vi "MTMount_getSample_Balancing.vi"(8 "error in (no error)":errorcluster, 11 "Balancing_Ctl":T1) -> (0 "error out":errorcluster, 2 "function return":i32, 3 "Balancing_Ctl out":T1)   [LabVIEW 2018, in "SALLV_MTMount.lvlib"]
doc: "int MTMount_shm_getSample_BalancingLV(MTMount_BalancingLV *Balancing_Ctl );"
uses:
  SALLV_MTMount.lvlib
  DataTypes/Balancing.ctl
  SALLV_MTMount.so
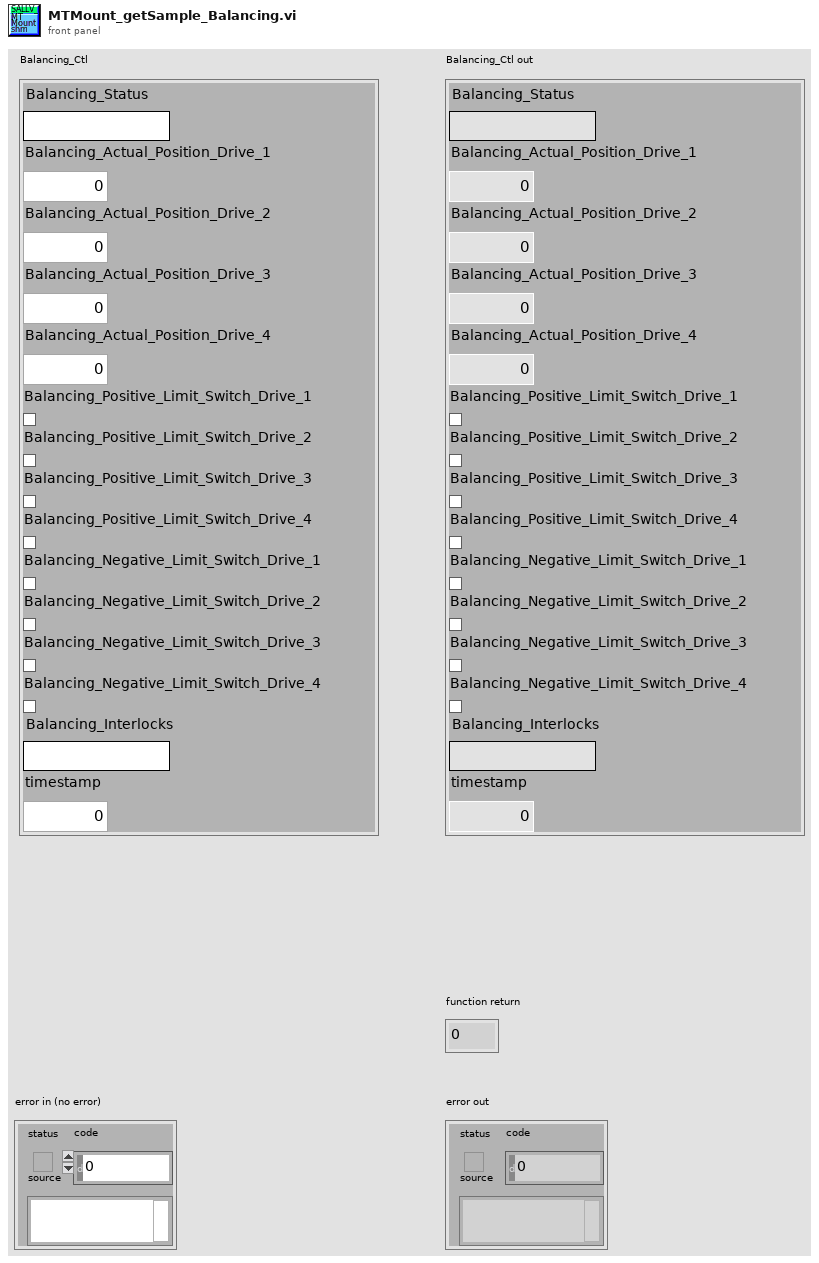
[diagram p1: front panel]
types:
  T1 = typedef "SALLV_MTMount.lvlib/Balancing.ctl" = cluster{"Balancing_Status":string, "Balancing_Actual_Position_Drive_1":dbl, "Balancing_Actual_Position_Drive_2":dbl, "Balancing_Actual_Position_Drive_3":dbl, "Balancing_Actual_Position_Drive_4":dbl, "Balancing_Positive_Limit_Switch_Drive_1":bool, "Balancing_Positive_Limit_Switch_Drive_2":bool, "Balancing_Positive_Limit_Switch_Drive_3":bool, "Balancing_Positive_Limit_Switch_Drive_4":bool, "Balancing_Negative_Limit_Switch_Drive_1":bool, "Balancing_Negative_Limit_Switch_Drive_2":bool, "Balancing_Negative_Limit_Switch_Drive_3":bool, "Balancing_Negative_Limit_Switch_Drive_4":bool, "Balancing_Interlocks":string, "timestamp":dbl}
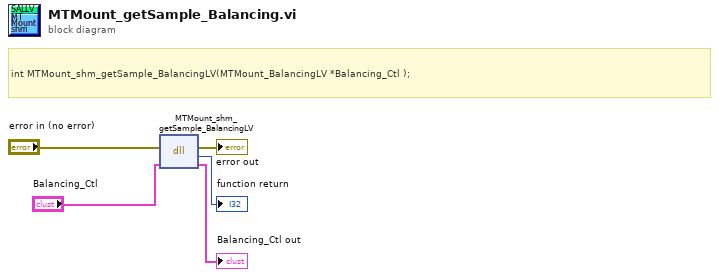
[diagram p0: block diagram]
diagram:
  # "int MTMount_shm_getSample_BalancingLV(MTMount_BalancingLV *Balancing_Ctl );"
  n1 = dll-call lib="home/ttsai/Document/salApiMTMount/SALLV_MTMount/SALLV_MTMount.*" fn="MTMount_shm_getSample_BalancingLV"(error in="error in (no error)", "Balancing_Ctl"="Balancing_Ctl") -> (error out=→"error out":errorcluster, →"function return":i32, "Balancing_Ctl"=→"Balancing_Ctl out":T1)  [unwired: 2 in, 1 out]
